vi "DFT Goertzel U16 1D.vi"(7 "ROI":T2, 8 "error in":errorcluster, 9 "DFT Settings":T3 {"Detrend"."Method" items=["Linear", "Quadratic", "Cubic", "N-polynomial", "Exponential", "None"]; "Window" items=["Rectangle"=0, "Hanning"=1, "Hamming"=2, "Blackman-Harris"=3, "Exact Blackman"=4, "Blackman"=5, "Flat Top"=6, "4 Term B-Harris "=7, "7 Term B-Harris"=8, "Low Sidelobe"=9, "Blackman Nuttall"=11, "Triangle"=30, "Bartlett-Hanning"=31, "Bohman"=32, "Parzen"=33, "Welch"=34, "Kaiser"=60, "Dolph-Chebyshev"=61, "Gaussian"=62]}, 10 "image array dims":T1, 11 "Images":u16[](array[numeric])) -> (0 "error out":errorcluster, 1 "FFT Bin":i32, 2 "Execution Time":u32, 3 "Analysis Cluster out":T5)   [LabVIEW 2023]
uses:
  <vilib>/Analysis/NI_AALPro.lvlib
  <vilib>/Analysis/NI_AALBase.lvlib
  <vilib>/Analysis/baseanly.llb/Scale 1D.vi
  <vilib>/Analysis/1siggen.llb/Ramp Pattern by Samples.vi
  DFT Settings.ctl
  <vilib>/Analysis/4window.llb/windowTd.ctl
panel:
  # "Execution Time 2400"
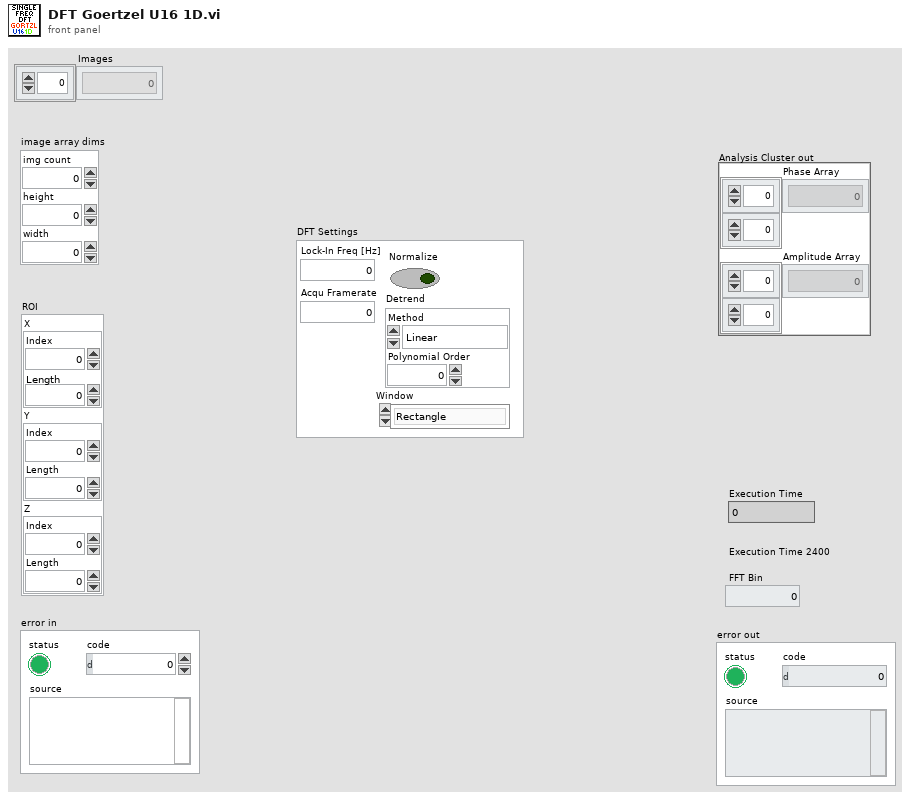
[diagram p1: front panel]
types:
  T1 = cluster{"img count":i32, "height":i32, "width":i32}
  T2 = cluster{"X":cluster{"Index":i32, "Length":i32}, "Y":cluster{"Index":i32, "Length":i32}, "Z":cluster{"Index":i32, "Length":i32}}
  T3 = typedef "tg-analysis.lvlib/DFT Settings.ctl" = cluster{"Lock-In Freq [Hz]":dbl, "Acqu Framerate":dbl, "Window":T4, "Detrend":cluster{"Method":u16, "Polynomial Order":i32}, "Normalize":bool}
  T4 = typedef "NI_AALPro.lvlib/windowTd.ctl" = u32
  T5 = cluster{"Phase Array":dbl[][], "Amplitude Array":dbl[][]}
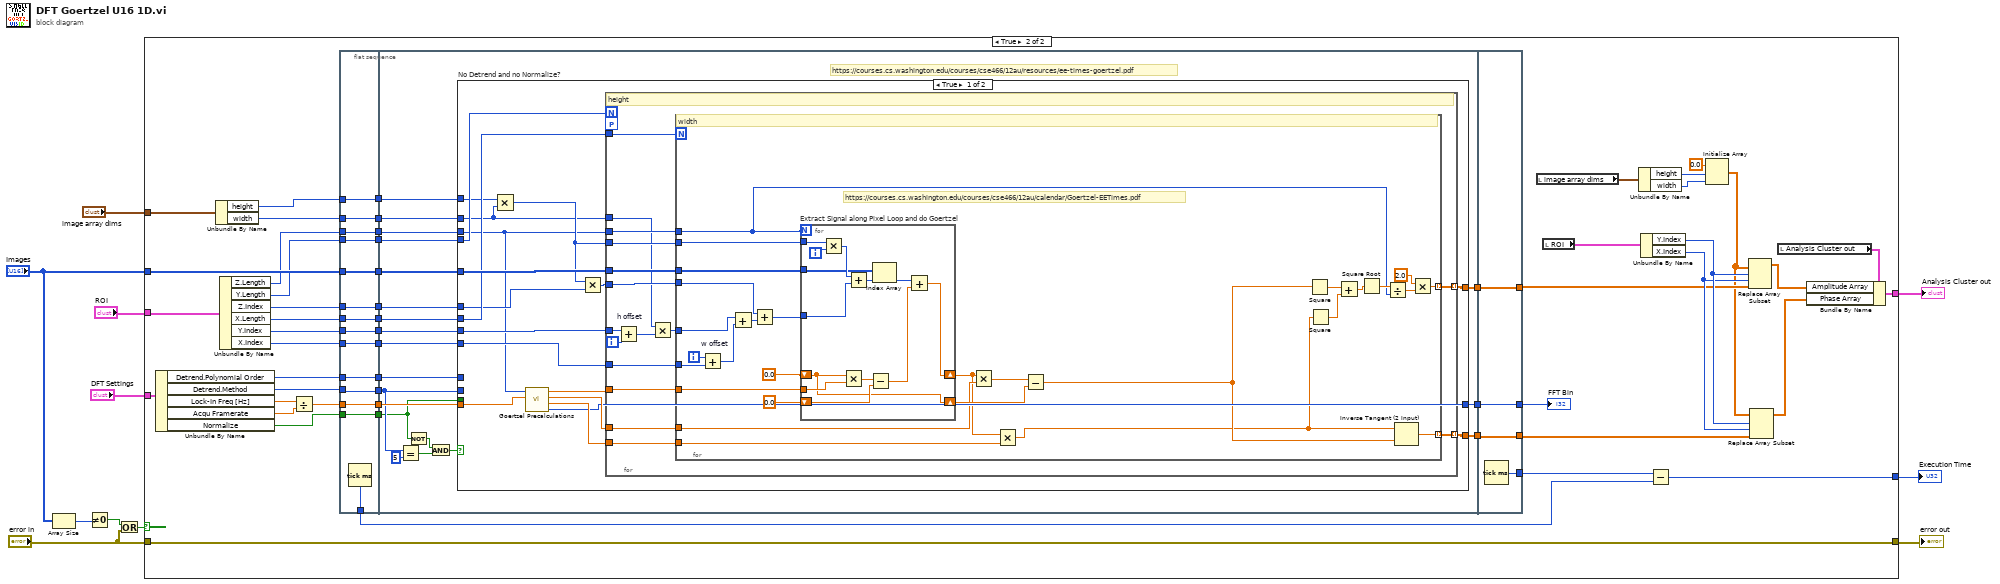
[diagram p0: block diagram]
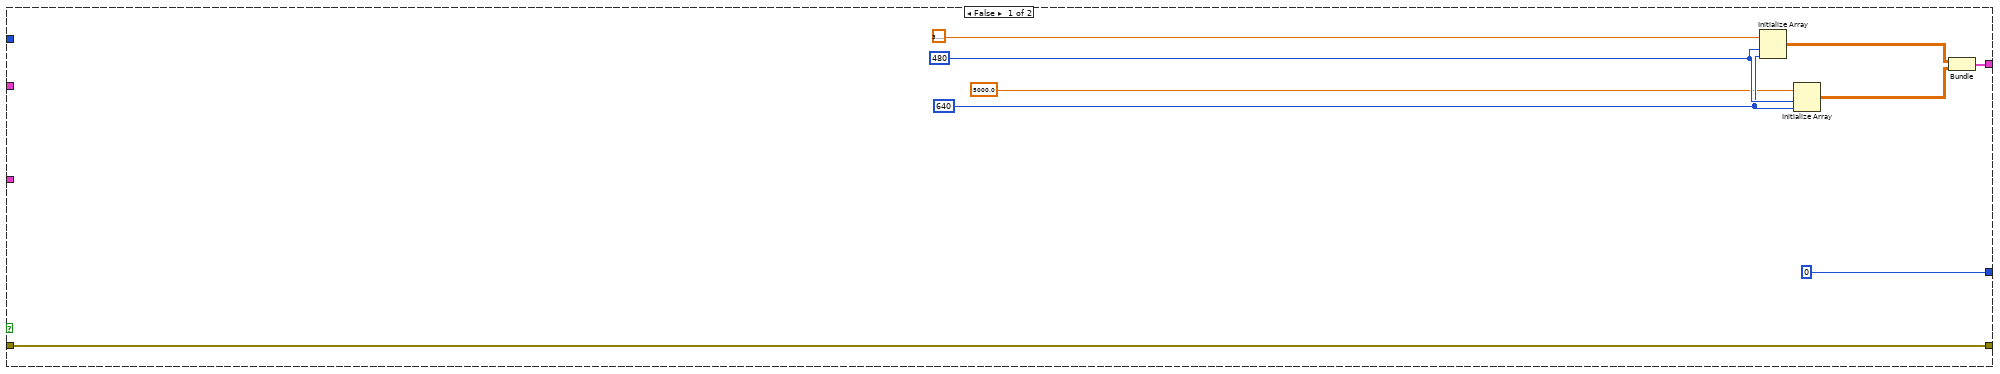
[diagram p2: hidden frame]
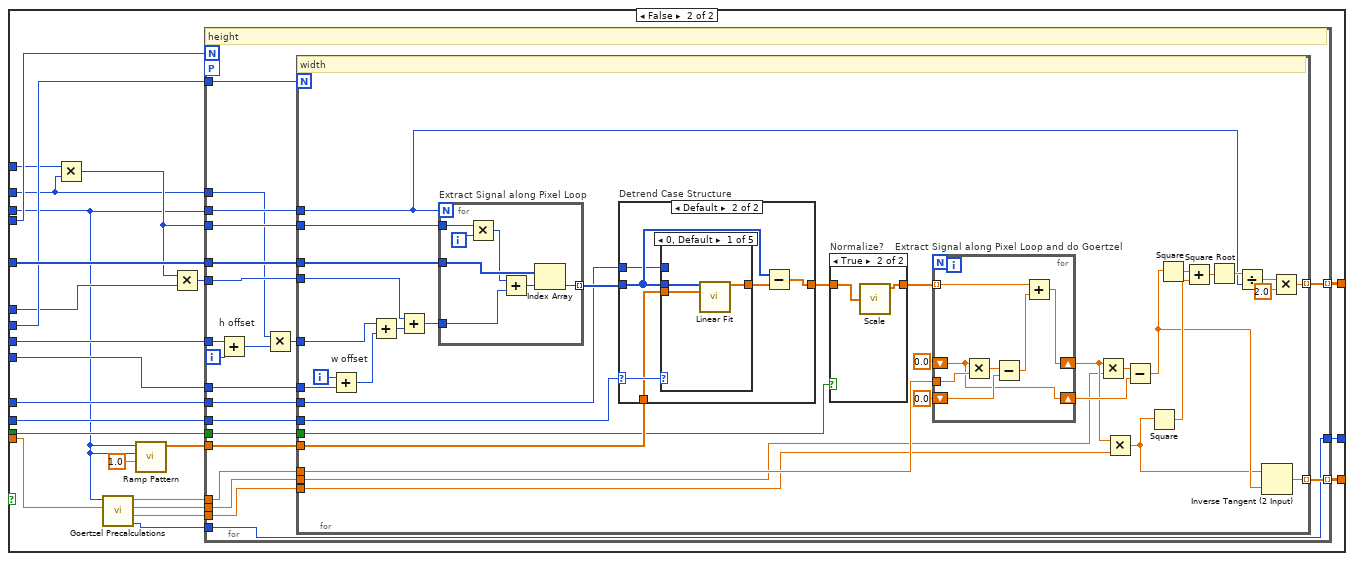
[diagram p3: hidden frame]
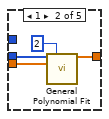
[diagram p6: hidden frame]
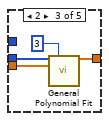
[diagram p7: hidden frame]
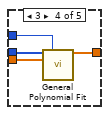
[diagram p8: hidden frame]
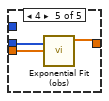
[diagram p9: hidden frame]
diagram:
  n1 = Array Size(array="Images") -> (size(s)=w2:i32)
  n2 = Not Equal To 0?(x=w2) -> (x != 0?=w5:bool)
  n3 = Or(x=w5, y="error in") -> (x .or. y?=w6:bool)
  n4 = case shown="True" w6 {
    tunnel: [u32 0 w73] -> w11
    tunnel: [w13 w57] -> w10
    tunnel: [w14 w70] -> w7
    tunnel: "Images" -> [_ w53]
    tunnel: "DFT Settings" -> [_ w62]
    tunnel: "ROI" -> [_ w59]
    tunnel: "error in" -> [w13 w57]
    tunnel: "image array dims" -> [_ w29]
    frame False {
      w18 = 640 ("dimension size")
      w19 = 480 ("dimension size")
      n5 = Initialize Array(3.141592653589793, w19, w18) -> (w16:dbl[][])
      n6 = Initialize Array(5000.0 ("element"), w19, w18) -> (w15:dbl[][])
      n7 = Bundle(w16, w15) -> (w14:cluster{dbl[][], dbl[][]})  [unwired: 1 in]
    }
    frame True {
      n8 = Unbundle By Name(w62) -> ("Detrend.Polynomial Order"=w61:i32, "Detrend.Method"=w60:u16, "Lock-In Freq [Hz]"=w56:dbl, "Acqu Framerate"=w55:dbl, "Normalize"=w25:bool)
      n9 = Unbundle By Name(w29) -> ("height"=w37:i32, "width"=w35:i32)
      n10 = Unbundle By Name(w59) -> ("Z.Length"=w32:i32, "Y.Length"=w33:i32, "Z.Index"=w30:i32, "X.Length"=w34:i32, "Y.Index"=w52:i32, "X.Index"=w51:i32)
      n11 = Divide(x=w56, y=w55) -> (x/y=w54:dbl)
      n12 = flat-sequence {
        tunnel: [w87] -> w41
        tunnel: w61 -> [w86]
        tunnel: [w86] -> w50
        tunnel: w60 -> [w85]
        tunnel: [w85] -> w49
        tunnel: w54 -> [w84]
        tunnel: [w84] -> w48
        tunnel: w53 -> [w83]
        tunnel: [w83] -> w47
        tunnel: w34 -> [w82]
        tunnel: [w82] -> w46
        tunnel: [w81] -> w45
        tunnel: w32 -> [w81]
        tunnel: [w80] -> w44
        tunnel: w52 -> [w80]
        tunnel: [w79] -> w43
        tunnel: w33 -> [w79]
        tunnel: [w78] -> w42
        tunnel: w51 -> [w78]
        tunnel: [w77] -> w38
        tunnel: w37 -> [w77]
        tunnel: [w76] -> w36
        tunnel: w35 -> [w76]
        tunnel: w30 -> [w75]
        tunnel: [w75] -> w31
        tunnel: [w74] -> w26
        tunnel: w25 -> [w74]
        tunnel: [w107] -> w72
        tunnel: [w106] -> w68
        tunnel: w36 -> [w97]
        tunnel: w38 -> [w98]
        tunnel: w42 -> [w99]
        tunnel: w43 -> [w103]
        tunnel: w44 -> [w104]
        tunnel: w45 -> [w96]
        tunnel: w46 -> [w101]
        tunnel: w47 -> [w102]
        tunnel: w48 -> [w94]
        tunnel: w49 -> [w93]
        tunnel: w50 -> [w105]
        tunnel: w31 -> [w100]
        tunnel: w26 -> [w88]
        tunnel: [w95] -> w24
        tunnel: [w308] -> w67
        tunnel: w72 -> [w308]
        tunnel: [w307] -> w71
        tunnel: w68 -> [w306]
        tunnel: [w306] -> w58
        tunnel: w24 -> [w305]
        tunnel: [w305] -> w23
        frame #0 {
          n13 = Tick Count (ms)() -> (millisecond timer value=w87:u32)
        }
        frame #1 {
          # "https://courses.cs.washington.edu/courses/cse466/12au/resources/ee-times-goertzel.pdf"
          n14 = Equal?(x=w93, y=u16 5) -> (x = y?=w91:bool)
          n15 = Not(x=w88) -> (.not. x?=w89:bool)
          n16 = And(x=w89, y=w91) -> (x .and. y?=w92:bool)
          n17 = case "No Detrend and no Normalize?" shown="True" w92 {
            tunnel: [w125 w206] -> w107
            tunnel: [w124 w205] -> w106
            tunnel: w105 -> [_ w204]
            tunnel: w93 -> [_ w203]
            tunnel: w104 -> [w123 w202]
            tunnel: w103 -> [w122 w201]
            tunnel: w102 -> [w121 w200]
            tunnel: w101 -> [w118 w197]
            tunnel: w100 -> [w117 w196]
            tunnel: w99 -> [w116 w195]
            tunnel: w98 -> [w115 w194]
            tunnel: w97 -> [w114 w193]
            tunnel: w88 -> [_ w191]
            tunnel: w96 -> [w113 w187]
            tunnel: [w108 w189] -> w95
            tunnel: w94 -> [w112 w188]
            frame True {
              n18 = Multiply(x=w115, y=w114) -> (x*y=w120:i32)
              n19 = call "Goertzel Precalculations.vi"("Cycles per Sample"=w112, "Sample Length"=w113) -> ("FFT Bin"=w108:i32, "Sine"=w109:dbl, "Cosine"=w110:dbl, "Coeff"=w111:dbl)  [unwired: 6 in]
              n20 = Multiply(x=w120, y=w117) -> (x*y=w119:i32)
              n21 = for "FT on rows Loop" {
                N: w122 -> [_]
                tunnel: [w141] -> w125 mode=indexing
                tunnel: [w139] -> w124 mode=indexing
                tunnel: w123 -> [w138]
                tunnel: w118 -> [w137]
                tunnel: w116 -> [w136]
                tunnel: w121 -> [w135]
                tunnel: w120 -> [w134]
                tunnel: w119 -> [w133]
                tunnel: w113 -> [w132]
                tunnel: w114 -> [w129]
                workers-P: _ -> [_]
                tunnel: w111 -> [w128]
                tunnel: w110 -> [w127]
                tunnel: w109 -> [w126]
                i -> [w140]
                # "height"
                n22 = Add "h offset"(x=w138, y=w140) -> (x+y=w131:i32)
                n23 = Multiply(x=w129, y=w131) -> (x*y=w130:i32)
                n24 = for "FT process cols Loop" {
                  N: w137 -> [_]
                  tunnel: [w148] -> w141 mode=indexing
                  tunnel: [w149] -> w139 mode=indexing
                  tunnel: w135 -> [w163]
                  tunnel: w136 -> [w168]
                  tunnel: w134 -> [w162]
                  tunnel: w133 -> [w165]
                  tunnel: w132 -> [w142]
                  tunnel: w130 -> [w164]
                  tunnel: w128 -> [w159]
                  tunnel: w127 -> [w146]
                  tunnel: w126 -> [w145]
                  i -> [w169]
                  # "https://courses.cs.washington.edu/courses/cse466/12au/calendar/Goertzel-EETimes.pdf"
                  # "width"
                  n25 = Add "w offset"(x=w169, y=w168) -> (x+y=w167:i32)
                  n26 = Add(x=w164, y=w167) -> (x+y=w166:i32)
                  n27 = Add(x=w165, y=w166) -> (x+y=w143:i32)
                  n28 = for "Extract Signal along Pixel Loop and do Goertzel" {
                    N: w142 -> [_]
                    tunnel: w163 -> [w177]
                    tunnel: w143 -> [w179]
                    tunnel: w162 -> [w181]
                    shift-right: [w170] -> w144
                    shift-left: 0.0 -> [w171]
                    tunnel: w159 -> [w176]
                    shift-right: [w171] -> w147
                    shift-left: 0.0 -> [w174]
                    i -> [w182]
                    n29 = Multiply(x=w181, y=w182) -> (x*y=w180:i32)
                    n30 = Multiply(x=w171, y=w176) -> (x*y=w175:dbl)
                    n31 = Add(x=w180, y=w179) -> (x+y=w178:i32)
                    n32 = Subtract(x=w175, y=w174) -> (x-y=w172:dbl)
                    n33 = Index Array(array=w177, index=w178) -> (element=w173:u16)
                    n34 = Add(x=w173, y=w172) -> (x+y=w170:dbl)
                  }
                  n35 = Multiply(x=w144, y=w146) -> (x*y=w154:dbl)
                  n36 = Multiply(x=w144, y=w145) -> (x*y=w152:dbl)
                  n37 = Subtract(x=w154, y=w147) -> (x-y=w153:dbl)
                  n38 = Square(x=w153) -> (x^2=w158:dbl)
                  n39 = Square(x=w152) -> (x^2=w157:dbl)
                  n40 = Add(x=w158, y=w157) -> (x+y=w156:dbl)
                  n41 = Square Root(x=w156) -> (sqrt(x)=w155:dbl)
                  n42 = Divide(x=w155, y=w142) -> (x/y=w151:dbl)
                  n43 = Inverse Tangent (2 Input)(1:w153, 2:w152) -> (0:w148:dbl)
                  n44 = Multiply(x=2.0, y=w151) -> (x*y=w149:dbl)
                }
              }
            }
            frame False {
              n45 = Multiply(x=w194, y=w193) -> (x*y=w199:i32)
              n46 = call "Goertzel Precalculations.vi"("Cycles per Sample"=w188, "Sample Length"=w187) -> ("FFT Bin"=w183:i32, "Sine"=w184:dbl, "Cosine"=w185:dbl, "Coeff"=w186:dbl)  [unwired: 6 in]
              n47 = call-poly <vilib>:"Ramp Pattern.vi"("start"=1.0, "end"=w187, "samples"=w187) -> ("Ramp Pattern"=w192:dbl[])  [unwired: 7 in, 1 out]
              n48 = Multiply(x=w199, y=w196) -> (x*y=w198:i32)
              n49 = for "FT on rows Loop" {
                N: w201 -> [_]
                tunnel: [w227] -> w206 mode=indexing
                tunnel: [w225] -> w205 mode=indexing
                tunnel: w204 -> [w224]
                tunnel: w203 -> [w223]
                tunnel: w202 -> [w222]
                tunnel: w197 -> [w221]
                tunnel: w195 -> [w220]
                tunnel: w200 -> [w219]
                tunnel: w199 -> [w218]
                tunnel: w198 -> [w217]
                tunnel: w187 -> [w216]
                tunnel: w193 -> [w213]
                workers-P: _ -> [_]
                tunnel: w192 -> [w212]
                tunnel: w191 -> [w211]
                tunnel: [w207] -> w189
                tunnel: w186 -> [w210]
                tunnel: w185 -> [w209]
                tunnel: w184 -> [w208]
                tunnel: w183 -> [w207]
                i -> [w226]
                # "height"
                n50 = Add "h offset"(x=w222, y=w226) -> (x+y=w215:i32)
                n51 = Multiply(x=w213, y=w215) -> (x*y=w214:i32)
                n52 = for "FT process cols Loop" {
                  N: w221 -> [_]
                  tunnel: [w261] -> w227 mode=indexing
                  tunnel: [w259] -> w225 mode=indexing
                  tunnel: w219 -> [w255]
                  tunnel: w224 -> [w248]
                  tunnel: w223 -> [w246]
                  tunnel: w220 -> [w257]
                  tunnel: w218 -> [w253]
                  tunnel: w217 -> [w251]
                  tunnel: w216 -> [w228]
                  tunnel: w214 -> [w250]
                  tunnel: w212 -> [w247]
                  tunnel: w211 -> [w245]
                  tunnel: w210 -> [w237]
                  tunnel: w209 -> [w236]
                  tunnel: w208 -> [w235]
                  i -> [w262]
                  # "width"
                  n53 = Add "w offset"(x=w262, y=w257) -> (x+y=w256:i32)
                  n54 = Add(x=w250, y=w256) -> (x+y=w254:i32)
                  n55 = Add(x=w251, y=w254) -> (x+y=w252:i32)
                  n56 = for "Extract Signal along Pixel Loop" {
                    N: w228 -> [_]
                    tunnel: w255 -> [w304]
                    tunnel: w252 -> [w300]
                    tunnel: w253 -> [w302]
                    tunnel: [w298] -> w249 mode=indexing
                    i -> [w303]
                    n57 = Multiply(x=w302, y=w303) -> (x*y=w301:i32)
                    n58 = Add(x=w301, y=w300) -> (x+y=w299:i32)
                    n59 = Index Array(array=w304, index=w299) -> (element=w298:u16)
                  }
                  n60 = case "Detrend Case Structure" shown="Default" w246 {
                    selector: w246 -> [_ w279]
                    tunnel: w249 -> [w273 w278]
                    tunnel: w248 -> [_ w277]
                    tunnel: [w273 w275] -> w244
                    tunnel: w247 -> [_ w274]
                    frame 5 {
                    }
                    frame Default {
                      n61 = case shown="0, Default" w279 {
                        tunnel: w278 -> [w282 w286 w289 w294 w297]
                        tunnel: w274 -> [w281 w284 w287 w293 w296]
                        tunnel: [w280 w285 w288 w292 w295] -> w276
                        tunnel: w277 -> [_ _ _ w291 _]
                        frame 0, Default {
                          n62 = call <vilib>:"Linear Fit.vi"("Y"=w282, "X"=w281) -> ("Best Linear Fit"=w280:dbl[])  [unwired: 4 in, 9 out]
                        }
                        frame 1 {
                          n63 = call <vilib>:"General Polynomial Fit.vi"("Y"=w286, "polynomial order"=2, "X"=w284) -> ("Best Polynomial Fit"=w285:dbl[])  [unwired: 9 in, 3 out]
                        }
                        frame 2 {
                          n64 = call <vilib>:"General Polynomial Fit.vi"("Y"=w289, "polynomial order"=3, "X"=w287) -> ("Best Polynomial Fit"=w288:dbl[])  [unwired: 9 in, 3 out]
                        }
                        frame 3 {
                          n65 = call <vilib>:"General Polynomial Fit.vi"("Y"=w294, "polynomial order"=w291, "X"=w293) -> ("Best Polynomial Fit"=w292:dbl[])  [unwired: 9 in, 3 out]
                        }
                        frame 4 {
                          n66 = call <vilib>:"Exponential Fit (obs).vi"("Y"=w297, "X"=w296) -> ("Best Exponential Fit"=w295:dbl[])  [unwired: 1 in, 4 out]
                        }
                      }
                      n67 = Subtract(x=w278, y=w276) -> (x-y=w275:dbl[])
                    }
                  }
                  n68 = case "Normalize?" shown="True" w245 {
                    tunnel: w244 -> [w270 w272]
                    tunnel: [w270 w271] -> w239
                    frame False {
                    }
                    frame True {
                      n69 = call-poly <vilib>:"Scale.vi"("X"=w272) -> ("Y=(X-offset)/scale"=w271:dbl[])  [unwired: 3 out]
                    }
                  }
                  n70 = for "Extract Signal along Pixel Loop and do Goertzel" {
                    tunnel: w239 -> [w263] mode=indexing
                    shift-right: [w264] -> w240
                    shift-left: 0.0 -> [w265]
                    tunnel: w237 -> [w269]
                    shift-right: [w265] -> w241
                    shift-left: 0.0 -> [w267]
                    n71 = Multiply(x=w265, y=w269) -> (x*y=w268:dbl)
                    n72 = Subtract(x=w268, y=w267) -> (x-y=w266:dbl)
                    n73 = Add(x=w263, y=w266) -> (x+y=w264:dbl)
                  }
                  n74 = Multiply(x=w240, y=w236) -> (x*y=w242:dbl)
                  n75 = Multiply(x=w240, y=w235) -> (x*y=w229:dbl)
                  n76 = Subtract(x=w242, y=w241) -> (x-y=w230:dbl)
                  n77 = Square(x=w229) -> (x^2=w233:dbl)
                  n78 = Square(x=w230) -> (x^2=w234:dbl)
                  n79 = Add(x=w234, y=w233) -> (x+y=w232:dbl)
                  n80 = Square Root(x=w232) -> (sqrt(x)=w231:dbl)
                  n81 = Divide(x=w231, y=w228) -> (x/y=w260:dbl)
                  n82 = Inverse Tangent (2 Input)(1:w230, 2:w229) -> (0:w261:dbl)
                  n83 = Multiply(x=w260, y=2.0) -> (x*y=w259:dbl)
                }
              }
            }
          }
        }
        frame #2 {
          n84 = Tick Count (ms)() -> (millisecond timer value=w307:u32)
        }
      }
      n85 = local read "image array dims"() -> (w22:T1)
      n86 = local read "ROI"() -> (w21:T2)
      n87 = Unbundle By Name(w22) -> ("height"=w28:i32, "width"=w27:i32)
      n88 = Unbundle By Name(w21) -> ("Y.Index"=w64:i32, "X.Index"=w63:i32)
      n89 = Subtract(x=w71, y=w41) -> (x-y=w73:u32)
      n90 = Initialize Array(0.0, w28, w27) -> (w39:dbl[][])
      n91 = Replace Array Subset(array=w39, new element=w58, index (row)=w64, index (col)=w63) -> (w65:dbl[][])
      n92 = Replace Array Subset(array=w39, new element=w67, index (row)=w64, index (col)=w63) -> (w66:dbl[][])
      n93 = local read "Analysis Cluster out"() -> (w69:T5)
      n94 = Bundle By Name(cluster=w69, "Amplitude Array"=w65, "Phase Array"=w66) -> (w70:T5)
      "FFT Bin" <- w23
    }
  }
  "Execution Time" <- w11
  "error out" <- w10
  "Analysis Cluster out" <- w7
